vi "Write ERD Dryer Example.vi"(0 "GEA Inputs":T3 {"Destination" format="%.0x"; "Source" format="%.0x"}, 1 "Read Timeout (ms)":u32=500, 2 "Device Selected":i32, 5 "Retry Count":i32=5, 11 "Error In":errorcluster, 13 "Verify ERD Response?":bool) -> (4 "Data Returned":string, 15 "Error Out":errorcluster)   [LabVIEW 2014]
doc: "This standalone VI reads the next message on the GEA2 bus OR waits until it receives a message with the command or data you specify. (.* = anything)"
uses:
  Common/LabVIEW GEA2 Toolkit/LabVIEW_GEA2_Toolkit.lvlibp/type defs/Source_Destination.ctl
  Common/LabVIEW GEA2 Toolkit/LabVIEW_GEA2_Toolkit.lvlibp/type defs/ERD Write Data In.ctl
  Common/LabVIEW GEA2 Toolkit/LabVIEW_GEA2_Toolkit.lvlibp/type defs/Data Type.ctl
  Common/LabVIEW GEA2 Toolkit/LabVIEW_GEA2_Toolkit.lvlibp
panel:
  in  "Write ERD List":T1[](array[typedef]) {"ERD Number" format="%.0x"}
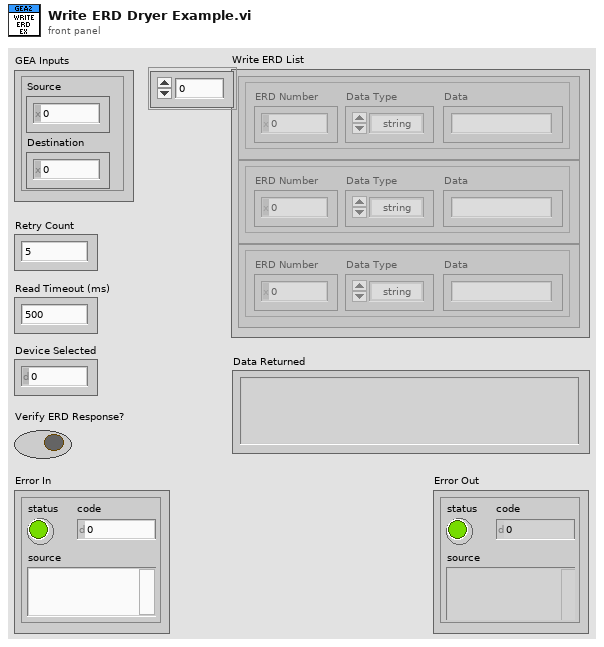
[diagram p1: front panel]
types:
  T1 = typedef "LabVIEW_GEA2_Toolkit.lvlibp/ERD Write Data In.ctl" = cluster{"ERD Number":u16, "Data Type":T2, "Data":string}
  T2 = typedef "LabVIEW_GEA2_Toolkit.lvlibp/Data Type.ctl" = enum16{"string", "boolean", "uint8_t", "uint16_t", "uint32_t", "uint64_t", "int8_t", "int16_t", "int32_t", "int64_t"}
  T3 = typedef "LabVIEW_GEA2_Toolkit.lvlibp/Source_Destination.ctl" = cluster{"Source":u8, "Destination":u8}
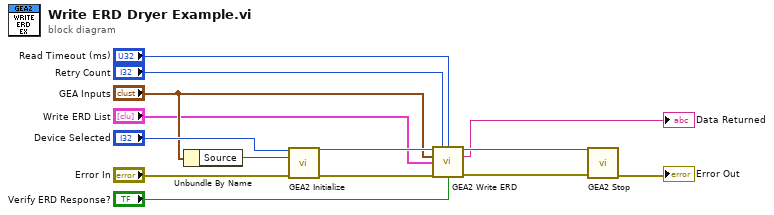
[diagram p0: block diagram]
diagram:
  n1 = Unbundle By Name("GEA Inputs") -> ("Source"=w2:u8)
  n2 = call "GEA2 Initialize.vi"("Board Index"="Device Selected", "Source Address"=w2, "error in"="Error In") -> ("GEA2 Reference Out"=w5:refnum<k24>, "error out"=w12:errorcluster)  [unwired: 10 in, 1 out]
  n3 = call "GEA2 Write ERD.vi"("GEA2 Reference In"=w5, "# of Tries"="Retry Count", "Read Timeout (ms)"="Read Timeout (ms)", "GEA Inputs"="GEA Inputs", "Write ERD List"="Write ERD List", "Error In"=w12, "Verify ERD Response?"="Verify ERD Response?") -> ("GEA2 Reference Out"=w13:refnum<k24>, "Raw Data Out"=→"Data Returned":string, "Error Out"=w14:errorcluster)  [unwired: 6 in]
  n4 = call "GEA2 Stop.vi"("GEA2 Reference In"=w13, "Error In"=w14) -> ("Error Out"=→"Error Out":errorcluster)  [unwired: 13 in]
